vi "Day13-2.vi"() -> ()   [LabVIEW 2021]
panel:
  out "Folded Paper":bool[][](array[boolean])
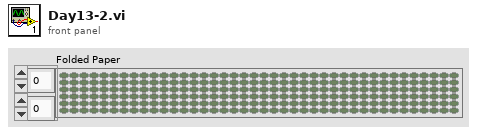
[diagram p1: front panel]
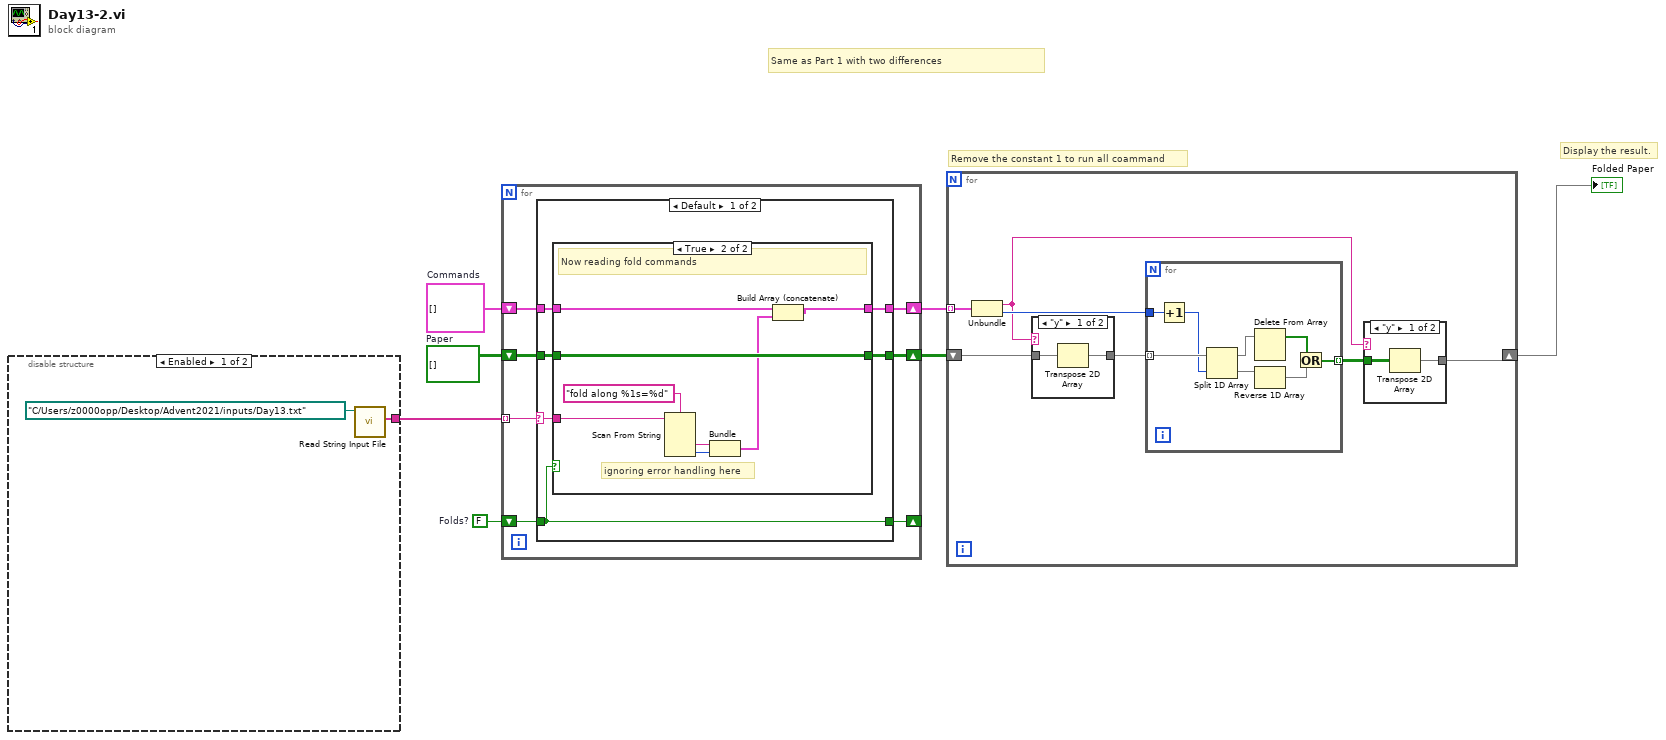
[diagram p0: block diagram]
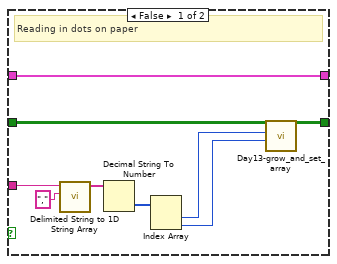
[diagram p4: hidden frame]
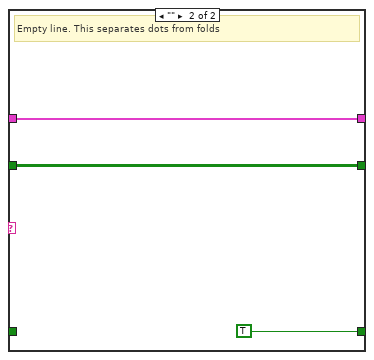
[diagram p5: hidden frame]
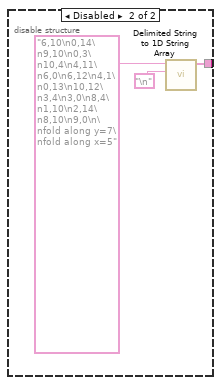
[diagram p6: hidden frame]
diagram:
  w4 = cluster{string, i32}[] []  # Commands
  w5 = bool[][] []  # Paper
  w6 = FALSE  # Folds?
  # "Same as Part 1 with two differences"
  # "Display the result."
  # "Remove the constant 1 to run all coammand"
  n1 = disable-structure shown="Enabled" {
    disable-tunnel: [w8 w10] -> w7
    frame Enabled {
      n2 = call "Read String Input File.vi"("file path (dialog if empty)"=path "C:/Users/z0000opp/Desktop/Advent2021/inputs/Day13.txt") -> ("input values"=w8:string[])  [unwired: 10 in]
    }
    frame Disabled {
      n3 = call <vilib>:"Delimited String to 1D String Array.vi"("delimiter"="\n", "delimited string"="6,10\n0,14\n9,10\n0,3\n10,4\n4,11\n6,0\n6,12\n4,1\n0,13\n10,12\n3,4\n3,0\n8,4\n1,10\n2,14\n8,10\n9,0\n\nfold along y=7\nfold along x=5") -> ("string array"=w10:string[])  [unwired: 9 in]
    }
  }
  n4 = for {
    tunnel: w7 -> [w19] mode=indexing
    shift-right: [w15] -> _
    shift-left: w6 -> [w18]
    shift-right: [w16] -> w2
    shift-left: w5 -> [w17]
    shift-right: [w13] -> w3
    shift-left: w4 -> [w14]
    n5 = case shown="Default" w19 {
      selector: w19 -> [w25 _]
      tunnel: w18 -> [w22 _]
      tunnel: w17 -> [w24 w45]
      tunnel: [w23 w45] -> w16
      tunnel: [w22 TRUE] -> w15
      tunnel: w14 -> [w21 w43]
      tunnel: [w20 w43] -> w13
      frame Default {
        n6 = case shown="True" w22 {
          tunnel: w25 -> [w34 w40]
          tunnel: w24 -> [w30 w42]
          tunnel: [w27 w42] -> w23
          tunnel: w21 -> [w26 w37]
          tunnel: [w26 w35] -> w20
          frame False {
            # "Reading in dots on paper"
            n7 = call <vilib>:"Delimited String to 1D String Array.vi"("delimiter"=",", "delimited string"=w34) -> ("string array"=w32:string[])  [unwired: 9 in]
            n8 = Decimal String To Number(string=w32) -> (number=w31:i32[])  [unwired: 2 in, 1 out]
            n9 = Index Array(array=w31) -> (element #1=w29:i32, element #2=w28:i32)  [unwired: 2 in]
            n10 = call "Day13-grow_and_set_array.vi"("row"=w28, "column"=w29, "Array in"=w30) -> ("Array out"=w27:bool[][])  [unwired: 8 in]
          }
          frame True {
            # "ignoring error handling here"
            # "Now reading fold commands"
            n11 = Scan From String(format string="fold along %1s=%d", input string=w40) -> (output 1=w39:string, output 2=w38:i32)  [unwired: 4 in, 3 out]
            n12 = Bundle(w39, w38) -> (w36:cluster{string, i32})  [unwired: 1 in]
            n13 = Build Array (concatenate)(w37, w36) -> (w35:cluster{string, i32}[])
          }
        }
      }
      frame "" {
        # "Empty line. This separates dots from folds"
      }
    }
  }
  n14 = for {
    tunnel: w3 -> [w52] mode=indexing
    shift-right: [w47] -> w1
    shift-left: w2 -> [w51]
    n15 = Unbundle(w52) -> (w46:string, w49:i32)
    n16 = case shown="\"y\"" w46 {
      tunnel: w51 -> [w65 w66]
      tunnel: [w64 w66] -> w50
      frame "y" {
        n17 = Transpose 2D Array(2D array=w65) -> (transposed array=w64:bool[][])
      }
      frame "x", Default {
      }
    }
    n18 = for {
      tunnel: w50 -> [w63] mode=indexing
      tunnel: w49 -> [w62]
      tunnel: [w56] -> w48 mode=indexing
      n19 = Increment(x=w62) -> (x+1=w61:i32)
      n20 = Split 1D Array(array=w63, index=w61) -> (first subarray=w60:bool[], second subarray=w59:bool[])
      n21 = Delete From Array(array=w60) -> (array with subset deleted=w57:bool[])  [unwired: 2 in, 1 out]
      n22 = Reverse 1D Array(array=w59) -> (reversed array=w58:bool[])
      n23 = Or(x=w57, y=w58) -> (x .or. y?=w56:bool[])
    }
    n24 = case shown="\"y\"" w46 {
      tunnel: w48 -> [w54 w55]
      tunnel: [w53 w55] -> w47
      frame "y" {
        n25 = Transpose 2D Array(2D array=w54) -> (transposed array=w53:bool[][])
      }
      frame "x", Default {
      }
    }
  }
  "Folded Paper" <- w1
